vi "SUBSTATUSCheck.vi"() -> (0 "Error 2":bool[](array[boolean]), 1 "No Errors":bool[](array[boolean]), 2 "Error":bool[](array[boolean]), 3 "No Errors":bool[](array[boolean]))   [LabVIEW 2021]
uses:
  <vilib>/Instr/_visa.llb/VISA Find Search Mode.ctl
  <vilib>/Instr/_visa.llb/VISA Configure Serial Port (Instr).vi
panel:
  out "unsigned byte array":u8[](array[numeric])
  out "Response":string
  out "find list":string[](array[string])
  out "read buffer 2":string
  in  "error in (no error) 3":errorcluster
  out "VISA resource name out 2":refnum<visa-resource-name>
  out "error out 2":errorcluster
  in  "error in (no error)":errorcluster
  out "error out":errorcluster
  out "VISA resource name out":refnum<visa-resource-name>
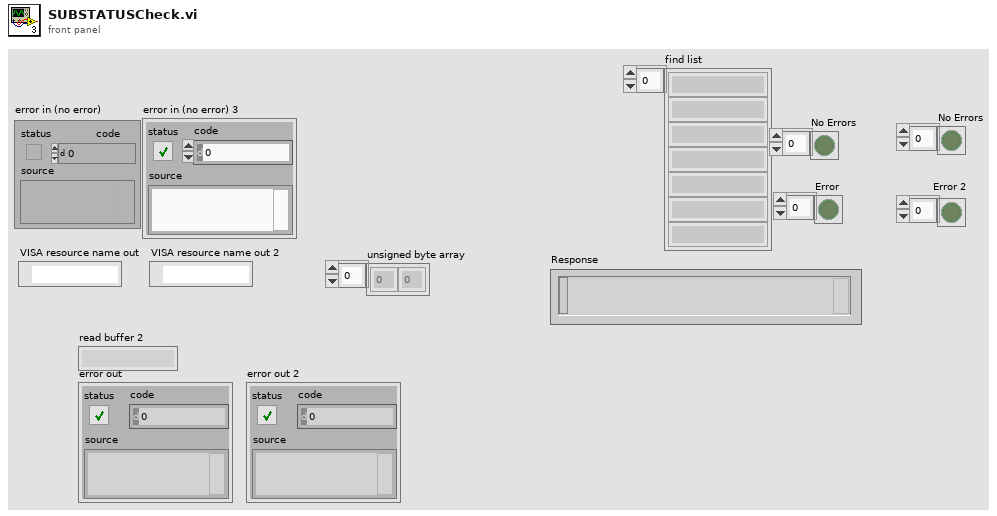
[diagram p1: front panel]
types:
  T1 = typedef "VISA Find Search Mode.ctl" = u32
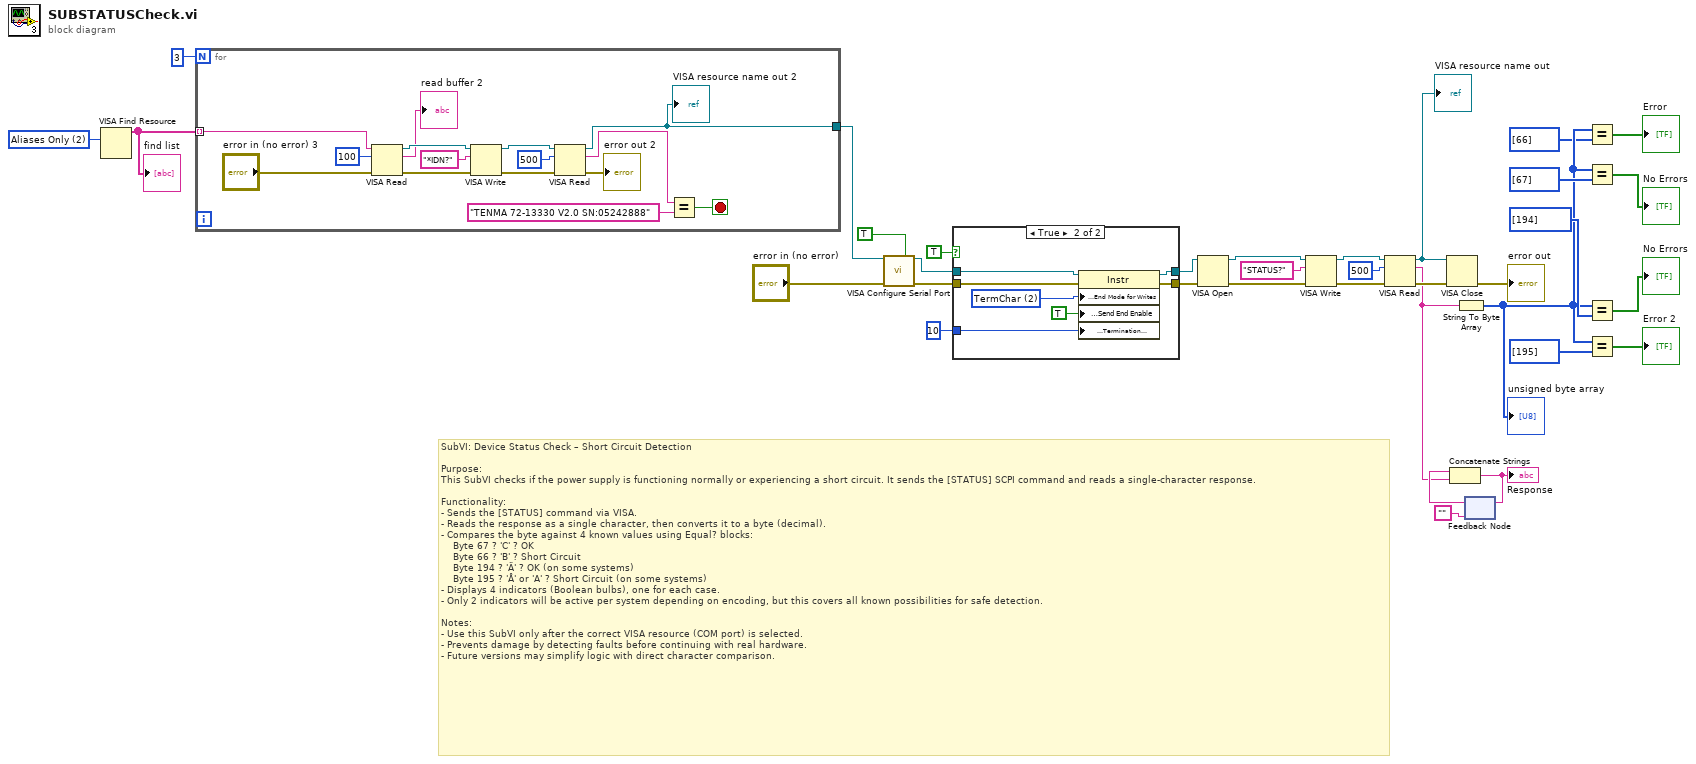
[diagram p0: block diagram]
diagram:
  w17 = T1 2 items=["Canonical Names Only"=0, "Aliases Only"=2, "Include Matching Aliases"=3, "Include All Aliases"=4] ("Search Mode")
  # "SubVI: Device Status Check – Short Circuit Detection\n\nPurpose:\nThis SubVI checks if the power supply is functioning normally or experiencing a short circuit. It sends the [STATUS] SCPI command and reads a single-character response.\n\nFunctionality:\n- Sends the [STATUS] command via VISA.\n- Reads the response as a single character, then converts it to a byte (decimal).\n- Compares the byte against 4 known values using Equal? blocks:\n    Byte 67 ? 'C' ? OK\n    Byte 66 ? 'B' ? Short Circuit\n    Byte 194 ? 'Ä' ? OK (on some systems)\n    Byte 195 ? 'Å' or 'A' ? Short Circuit (on some systems)\n- Displays 4 indicators (Boolean bulbs), one for each case.\n- Only 2 indicators will be active per system depending on encoding, but this covers all known possibilities for safe detection.\n\nNotes:\n- Use this SubVI only after the correct VISA resource (COM port) is selected.\n- Prevents damage by detecting faults before continuing with real hardware.\n- Future versions may simplify logic with direct character comparison."
  n1 = VISA Find Resource(10:w17) -> (3:w16:string[])  [unwired: 2 in, 2 out]
  "find list" <- w16
  n2 = for {
    N: 3 -> [_]
    tunnel: w16 -> [w49] mode=indexing
    tunnel: [w38] -> w15
    stop <- w42 stop-if-true
    n3 = VISA Read(VISA resource name=w49, byte count=u32 100, error in (no error)="error in (no error) 3") -> (VISA resource name out=w44:refnum<visa-resource-name>, read buffer=→"read buffer 2":string, error out=w39:errorcluster)  [unwired: 1 out]
    n4 = VISA Write(VISA resource name=w44, write buffer="*IDN?", error in (no error)=w39) -> (VISA resource name out=w47:refnum<visa-resource-name>, error out=w41:errorcluster)  [unwired: 1 out]
    n5 = VISA Read(VISA resource name=w47, byte count=u32 500, error in (no error)=w41) -> (VISA resource name out=w38:refnum<visa-resource-name>, read buffer=w45:string, error out=→"error out 2":errorcluster)  [unwired: 1 out]
    "VISA resource name out 2" <- w38
    n6 = Equal?(x=w45, y="TENMA 72-13330 V2.0 SN:05242888") -> (x = y?=w42:bool)
  }
  n7 = call-poly "VISA Configure Serial Port"("VISA resource name"=w15, "Enable Termination\nChar (T)"=TRUE ("End Read on Termination Character?"), "error in (no error)"="error in (no error)") -> ("VISA resource name out"=w22:refnum<visa-resource-name>, "error out"=w21:errorcluster)  [unwired: 7 in, 4 out]
  n8 = case shown="True" TRUE ("End Write on Termination Character?") {
    tunnel: w22 -> [w50 w58]
    tunnel: w21 -> [w51 w57]
    tunnel: [w50 w56] -> w20
    tunnel: [w51 w55] -> w19
    tunnel: u8 10 ("Termination Character") -> [_ w53]
    frame False {
    }
    frame True {
      w54 = u16 2 items=["None", "LastBit", "TermChar", "Break"] ("Serial Settings:Serial End Mode for Writes")
      n9 = property class="Instr"(reference=w58, error in=w57, "Serial Settings:End Mode for Writes"=w54, "Message Based Settings:Send End Enable"=TRUE, "Message Based Settings:Termination Character"=w53) -> (reference out=w56:refnum<visa-resource-name>, error out=w55:errorcluster)
    }
  }
  n10 = VISA Open(error in (no error)=w19, VISA resource name=w20) -> (VISA resource name=w34:refnum<visa-resource-name>, error out=w32:errorcluster)  [unwired: 3 in]
  n11 = VISA Write(VISA resource name=w34, write buffer="STATUS?", error in (no error)=w32) -> (VISA resource name out=w31:refnum<visa-resource-name>, error out=w29:errorcluster)  [unwired: 1 out]
  n12 = VISA Read(VISA resource name=w31, byte count=u32 500, error in (no error)=w29) -> (VISA resource name out=w28:refnum<visa-resource-name>, read buffer=w10:string, error out=w27:errorcluster)  [unwired: 1 out]
  "VISA resource name out" <- w28
  n13 = VISA Close(VISA resource name=w28, error in (no error)=w27) -> (error out=→"error out":errorcluster)
  n14 = String To Byte Array(string=w10) -> (unsigned byte array=w3:u8[])
  "unsigned byte array" <- w3
  n15 = feedback #1("") -> (w13:string)
  n16 = Concatenate Strings(w13, w10) -> (w12:string)
  "Response" <- w12
  n17 = feedback-in #1(w12) -> ()
  n18 = Equal?(x=w3, y=u8[] [66]) -> (x = y?=→"Error":bool[])
  n19 = Equal?(x=w3, y=u8[] [67] ("unsigned byte array")) -> (x = y?=→"No Errors":bool[])
  n20 = Equal?(x=w3, y=u8[] [194]) -> (x = y?=→"No Errors":bool[])
  n21 = Equal?(x=w3, y=u8[] [195]) -> (x = y?=→"Error 2":bool[])
